vi "PrefDialog.vi"(8 "error in (no error)":errorcluster, 11 "MyPluginsBase in":refnum<class "NiDaqMx.lvclass">) -> (0 "error out":errorcluster, 3 "MyPluginsBase out":refnum<class "NiDaqMx.lvclass">)   [LabVIEW 2018, in "DigitizerPlugins.lvlib" / "NiDaqMx.lvclass"]
uses:
  NiDaqMx.lvclass
  X:/Projects/PMUCal/Modules/Digitizer/DigitizerPlugins/DigitizerBaseClass/DigitizerBase.lvclass
  C:/Program Files (x86)/National Instruments/LabVIEW 2018/user.lib/NIST/BaseClasses/BasePlugin_class/BasePlugin.lvclass
  DigitizerBaseClass/Typedefs/Acquisition.ctl
  DigitizerBaseClass/Typedefs/Channel.ctl
  DigitizerBaseClass/Typedefs/Trigger.ctl
  DigitizerBaseClass/Typedefs/TrigSource.ctl
  SampleClock.ctl
  Typedefs/Sync.ctl
  Typedefs/ExportSignal.ctl
  DigitizerBaseClass/DigitizerBase.lvclass/DigitizerBase.ctl
  NiDaqMx.lvclass/NiDaqMx.ctl
  <userlib>/NIST/BaseClasses/BasePlugin_class/BasePlugin.lvclass/BasePlugin.ctl
  DigitizerBaseClass/Accessors/Read Acquisition.vi
  DigitizerBaseClass/Accessors/Read Trigger.vi
  DigitizerBaseClass/Accessors/Read Channels.vi
  Accessors/Read SampleClock.vi
  Accessors/Read ExportSignal.vi
  DigitizerBaseClass/Accessors/Read SyncInfo.vi
  <userlib>/NIST/BaseClasses/BasePlugin_class/Accessors/Read PluginIniFilePath.vi
  DigitizerBaseClass/Accessors/Write Acquisition.vi
  DigitizerBaseClass/Accessors/Write Trigger.vi
  DigitizerBaseClass/Accessors/Write Channels.vi
  Accessors/Write SampleClock.vi
  DigitizerBaseClass/Accessors/Write SyncInfo.vi
  Accessors/Write ExportSignal.vi
  <userlib>/NIST/BaseClasses/BasePlugin_class/Accessors/Write PluginIniFilePath.vi
  <vilib>/Utility/config.llb/NI_LVConfig.lvlib
  DigitizerBaseClass/DigitizerBase.lvclass
panel:
  in  "cntrlTab":T1(tab)
  in  "Channels":T2[](array[typedef])
  in  "Acquisition":T3 {"SampleMode" items=["Real Time", "Equivalent Time"]}
  in  "Trigger":T4
  in  "ExportSignal":T6={"signal"=12487, "Destination"="none", "Route"="none"} {"signal" items=["AI Convert Clock"=12484, "10MHz Reference Clock"=12536, "20MHz Timebase Clock"=12486, "Sample Clock"=12487, "Advance Trigger"=12488, "Reference Trigger"=12490, "Start Trigger"=12491, "Advance Complete Event"=12492, "AI Hold Complete Event"=12493, "Counter Output Event"=12494, "Change Detection Event"=12511, "Watchdog Timer Expired Event"=12512]}
  in  "SampleClock":T7 {"sample mode" items=["Finite Samples"=10178, "Continuous Samples"=10123, "Hardware Timed Single Point"=12522]; "TimebaseRate" format="%#_6p"}
  in  "Sync":T8
  in  "btnSaveAs":bool
  in  "btnSave":bool
  in  "btnCancel":bool
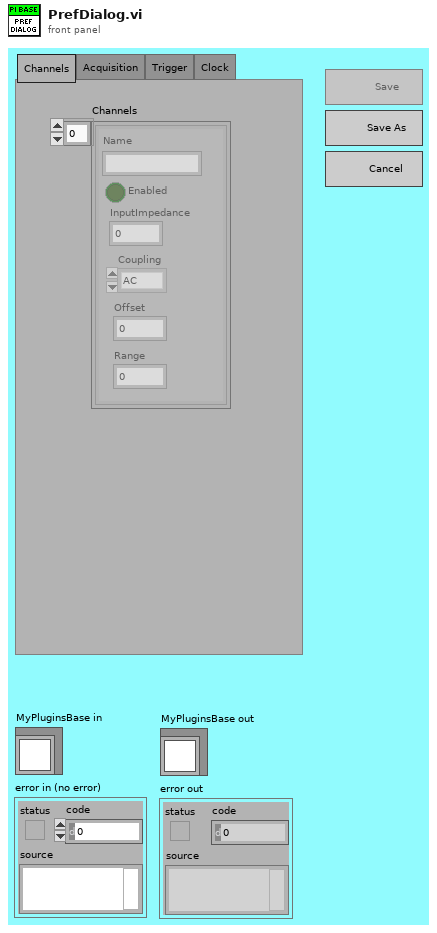
[diagram p1: front panel]
types:
  T1 = enum32{"Channels", "Acquisition", "Trigger", "Clock"}
  T2 = typedef "DigitizerPlugins.lvlib/DigitizerBase.lvclass/Channel.ctl" = cluster{"Name":string, "Enabled":bool, "InputImpedance":dbl, "Coupling":enum16{"AC", "DC", "Gnd"}, "Offset":dbl, "Range":dbl}
  T3 = typedef "DigitizerPlugins.lvlib/DigitizerBase.lvclass/Acquisition.ctl" = cluster{"SampleRate":dbl, "RecordSize":i32, "NumRecords":i32, "SampleMode":i32, "Timeout (ms)":i32}
  T4 = typedef "DigitizerPlugins.lvlib/DigitizerBase.lvclass/Trigger.ctl" = cluster{"Source":string, "Delay":dbl, "Holdoff":dbl, "PretriggerSamples":i32, "Sources":T5[]}
  T5 = typedef "DigitizerPlugins.lvlib/DigitizerBase.lvclass/TrigSource.ctl" = cluster{"Name":string, "Coupling":enum16{"AC", "DC", "HF Reject", "LF Reject", "Noise Reject"}, "Hysteresis":dbl, "Level":dbl, "Slope":enum16{"Positive", "Negative"}, "Type":enum16{"Edge", "Width", "Runt", "Glitch", "TV", "Window"}}
  T6 = typedef "DigitizerPlugins.lvlib/NiDaqMx.lvclass/ExportSignal.ctl" = cluster{"signal":i32, "Destination":string, "Route":string}
  T7 = typedef "DigitizerPlugins.lvlib/NiDaqMx.lvclass/SampleClock.ctl" = cluster{"Type":enum16{"NULL", "Onboard", "External", "Software", "Interval"}, "Source":string, "TimebaseRate":dbl, "sample mode":i32}
  T8 = typedef "DigitizerPlugins.lvlib/NiDaqMx.lvclass/Sync.ctl" = cluster{"Handle":string, "SrcTerm":string, "DestTerm":string}
  T9 = enum32{"Invalid", "Default", "Floating", "Floating/Auto-Hide", "Modal"}
  T10 = enum8{"Enabled", "Disabled", "Disabled and Grayed Out"}
  T11 = typedef "NI_LVConfig.lvlib/Config Data RefNum.ctl" = refnum<k1>
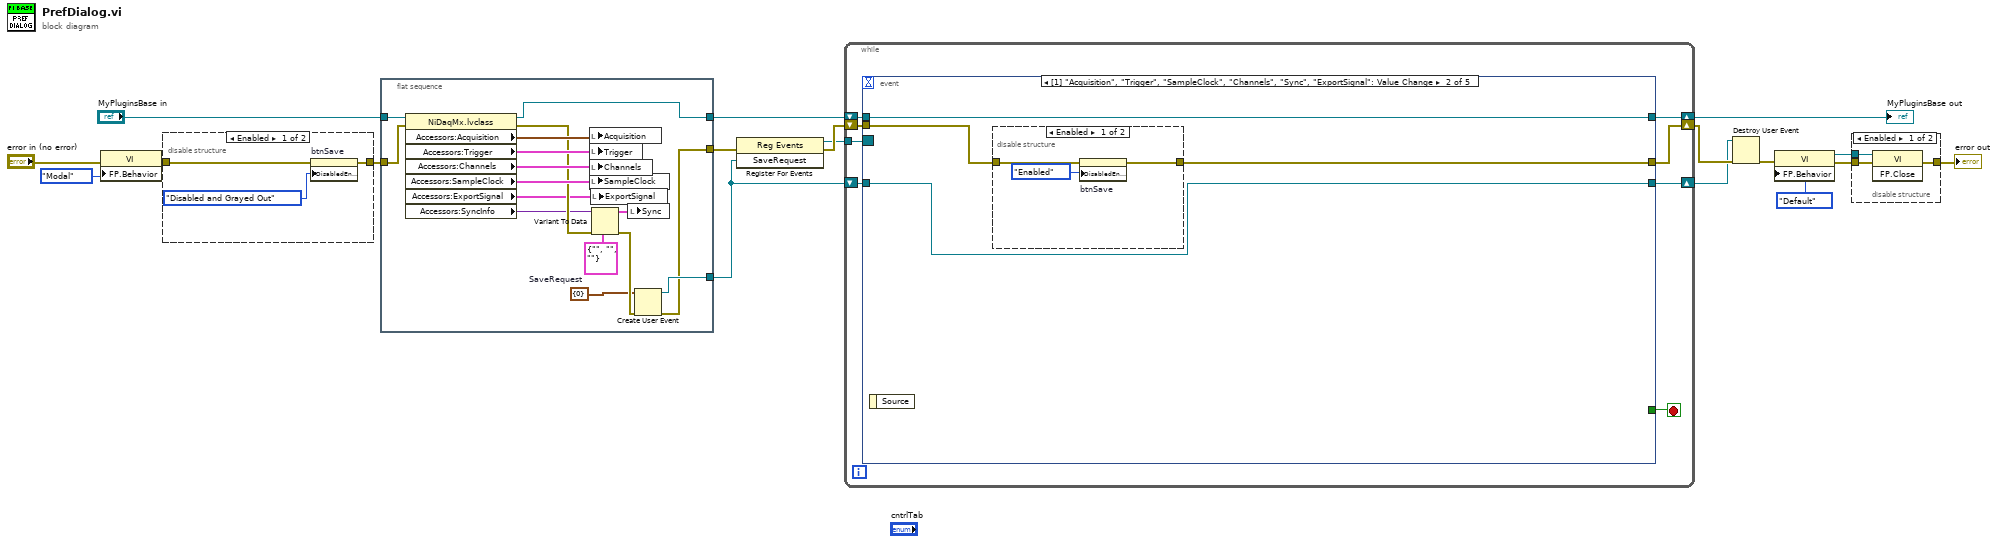
[diagram p0: block diagram]
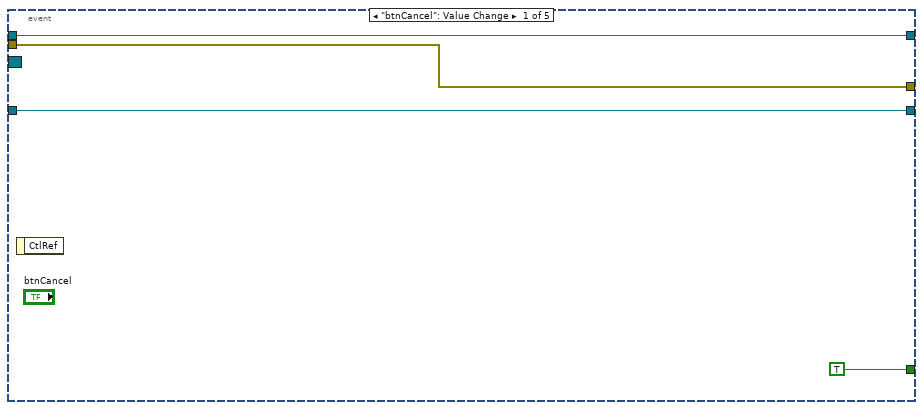
[diagram p4: hidden frame]
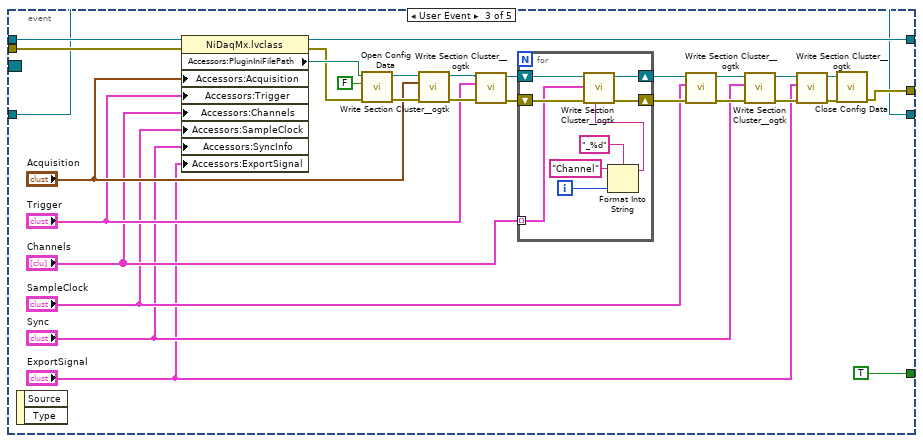
[diagram p6: hidden frame]
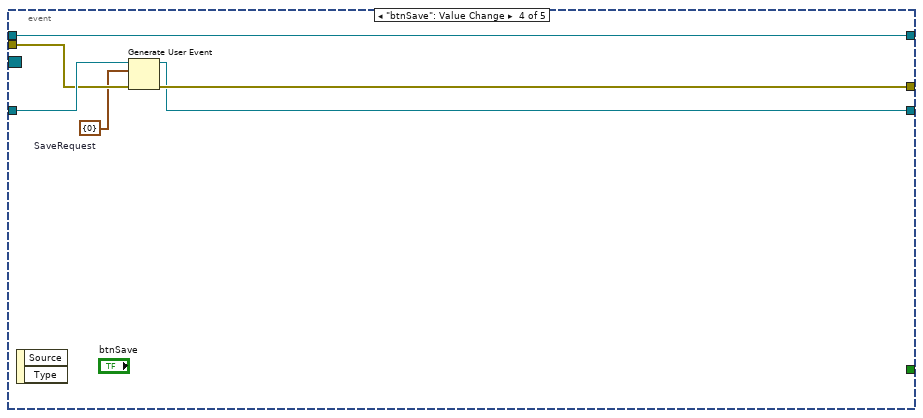
[diagram p7: hidden frame]
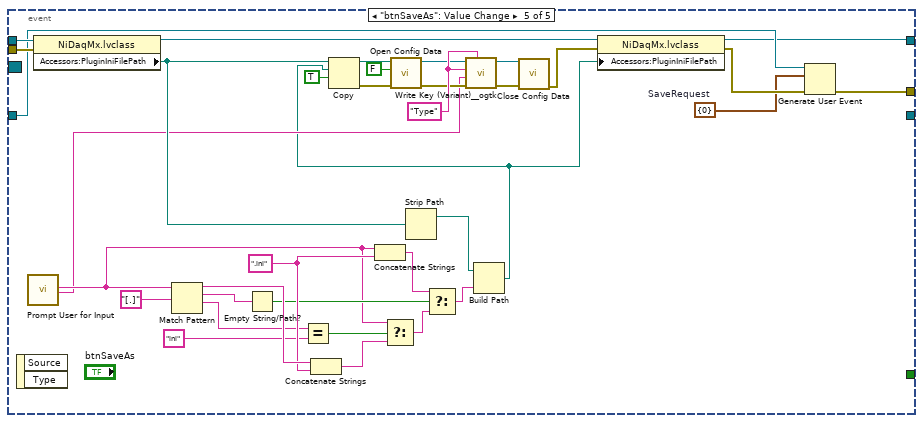
[diagram p8: hidden frame]
diagram:
  n1 = property class="VI"(error in="error in (no error)", "FP.Behavior"=T9."Modal" ("Front Panel Window:Behavior")) -> (error out=w9:errorcluster)  [unwired: 1 in, 1 out]
  n2 = disable-structure shown="Enabled" {
    disable-tunnel: w9 -> [w20 w22]
    disable-tunnel: [w19 w22] -> w8
    frame Enabled {
      n3 = property on="btnSave" class="Bool"(error in=w20, "DisabledEnum"=T10."Disabled and Grayed Out" ("Disabled")) -> (error out=w19:errorcluster)  [unwired: 1 in, 1 out]
    }
    frame Disabled {
    }
  }
  n4 = flat-sequence {
    tunnel: "MyPluginsBase in" -> [w38]
    tunnel: [w32] -> w10
    tunnel: [w25] -> w7
    tunnel: w8 -> [w30]
    tunnel: [w27] -> w2
    frame #0 {
      w24 = cluster{"num":i32} {"num"=0}  # SaveRequest
      n5 = property class="NiDaqMx.lvclass"(reference=w38, error in=w30) -> (reference out=w32:refnum<class "NiDaqMx.lvclass">, error out=w33:errorcluster, "Accessors:Acquisition"=w37:T3, "Accessors:Trigger"=w36:T4, "Accessors:Channels"=w35:T2[], "Accessors:SampleClock"=w34:T7, "Accessors:ExportSignal"=w23:T6, "Accessors:SyncInfo"=w31:variant)
      n6 = local write "Acquisition"(w37) -> ()
      n7 = local write "Trigger"(w36) -> ()
      n8 = local write "Channels"(w35) -> ()
      n9 = local write "SampleClock"(w34) -> ()
      n10 = local write "ExportSignal"(w23) -> ()
      n11 = Variant To Data(error in=w33, type=T8 {"Handle"="", "SrcTerm"="", "DestTerm"=""} ("Sync"), Variant=w31) -> (data=w28:T8, error out=w26:errorcluster)
      n12 = local write "Sync"(w28) -> ()
      n13 = Create User Event(user event datatype=w24, error in=w26) -> (user event=w27:refnum<user-event>, error out=w25:errorcluster)
    }
  }
  n14 = register-events(error in=w7, w2) -> (reference out=w5:refnum<event-registration>, error out=w6:errorcluster)  [unwired: 1 in]
  n15 = while {
    shift-right: [w46] -> w18
    shift-left: w10 -> [w44]
    shift-right: [w45] -> w3
    shift-left: w6 -> [w43]
    tunnel: w5 -> [w41]
    shift-right: [w39] -> w1
    shift-left: w2 -> [w40]
    stop <- w42 stop-if-true
    n16 = event shown="[1] \"Acquisition\", \"Trigger\", \"SampleClock\", \"Channels\", \"Sync\", \"ExportSignal\": Value Change" {
      selector: w41 -> [_ _ _ _ _]
      dyn-events: _ -> [_ _ _ _ _]
      timeout: _ -> [_ _ _ _ _]
      tunnel: w44 -> [w50 w54 w87 w98 w124]
      tunnel: [w50 w54 w74 w98 w103] -> w46
      tunnel: [w49 w52 w73 w99 w104] -> w45
      tunnel: w43 -> [w49 w53 w86 w101 w123]
      tunnel: [TRUE _ TRUE _ _] -> w42
      tunnel: w40 -> [w47 w51 w59 w102 w107]
      tunnel: [w47 w51 w59 w97 _] -> w39
      event "btnCancel": Value Change {
        n17 = event-data() -> ()  [unwired: 1 in, 1 out]
      }
      event "Channels": Value Change {
        n18 = event-data() -> ()  [unwired: 1 in, 1 out]
        n19 = disable-structure shown="Enabled" {
          disable-tunnel: w53 -> [w57 w58]
          disable-tunnel: [w56 w58] -> w52
          frame Enabled {
            n20 = property on="btnSave" class="Bool"(error in=w57, "DisabledEnum"=T10."Enabled" ("Disabled")) -> (error out=w56:errorcluster)  [unwired: 1 in, 1 out]
          }
          frame Disabled {
          }
        }
      }
      event User Event {
        n21 = event-data() -> ()  [unwired: 1 in, 2 out]
        n22 = property class="NiDaqMx.lvclass"(reference=w87, error in=w86, "Accessors:Acquisition"="Acquisition", "Accessors:Trigger"="Trigger", "Accessors:Channels"="Channels", "Accessors:SampleClock"="SampleClock", "Accessors:SyncInfo"="Sync", "Accessors:ExportSignal"="ExportSignal") -> (reference out=w74:refnum<class "NiDaqMx.lvclass">, error out=w83:errorcluster, "Accessors:PluginIniFilePath"=w85:path)
        n23 = call <vilib>:"Open Config Data.vi"("error in (no error)"=w83, "create file if necessary (T)"=FALSE, "configuration file path"=w85) -> ("error out"=w81:errorcluster, "refnum"=w82:T11)  [unwired: 6 in, 1 out]
        n24 = call <userlib>:"Write Section Cluster__ogtk.vi"("error in (no error)"=w81, "Section Formatted Cluster"="Acquisition", "refnum"=w82) -> ("error out"=w79:errorcluster, "dup refnum"=w80:T11)  [unwired: 7 in]
        n25 = call <userlib>:"Write Section Cluster__ogtk.vi"("error in (no error)"=w79, "Section Formatted Cluster"="Trigger", "refnum"=w80) -> ("error out"=w78:errorcluster, "dup refnum"=w77:T11)  [unwired: 7 in]
        n26 = for {
          shift-right: [w94] -> w76
          shift-left: w78 -> [w96]
          shift-right: [w93] -> w75
          shift-left: w77 -> [w95]
          tunnel: "Channels" -> [w89] mode=indexing
          i -> [w90]
          n27 = Format Into String(format string="_%d", initial string="Channel", w90) -> (resulting string=w88:string)  [unwired: 1 in, 1 out]
          n28 = call <userlib>:"Write Section Cluster__ogtk.vi"("section (optional)"=w88, "error in (no error)"=w96, "Section Formatted Cluster"=w89, "refnum"=w95) -> ("error out"=w94:errorcluster, "dup refnum"=w93:T11)  [unwired: 6 in]
        }
        n29 = call <userlib>:"Write Section Cluster__ogtk.vi"("error in (no error)"=w76, "Section Formatted Cluster"="SampleClock", "refnum"=w75) -> ("error out"=w68:errorcluster, "dup refnum"=w67:T11)  [unwired: 7 in]
        n30 = call <userlib>:"Write Section Cluster__ogtk.vi"("error in (no error)"=w68, "Section Formatted Cluster"="Sync", "refnum"=w67) -> ("error out"=w62:errorcluster, "dup refnum"=w61:T11)  [unwired: 7 in]
        n31 = call <userlib>:"Write Section Cluster__ogtk.vi"("error in (no error)"=w62, "Section Formatted Cluster"="ExportSignal", "refnum"=w61) -> ("error out"=w64:errorcluster, "dup refnum"=w63:T11)  [unwired: 7 in]
        n32 = call <vilib>:"Close Config Data.vi"("error in (no error)"=w64, "refnum"=w63) -> ("error out"=w73:errorcluster)  [unwired: 8 in, 1 out]
      }
      event "btnSave": Value Change {
        w100 = cluster{i32} {0}  # SaveRequest
        n33 = event-data() -> ()  [unwired: 1 in, 2 out]
        n34 = Generate User Event(user event=w102, event data cluster=w100, error in=w101) -> (user event out=w97:refnum<user-event>, error out=w99:errorcluster)  [unwired: 1 in]
      }
      event "btnSaveAs": Value Change {
        w105 = cluster{i32} {0}  # SaveRequest
        w120 = "Type" ("key (optional)")
        w135 = ".ini" ("string")
        n35 = event-data() -> ()  [unwired: 1 in, 2 out]
        n36 = call "Prompt User for Input"() -> ("File Name"=w126:string, "PluginType"=w111:string)  [unwired: 16 in, 2 out]
        n37 = property class="NiDaqMx.lvclass"(reference=w124, error in=w123) -> (reference out=w110:refnum<class "NiDaqMx.lvclass">, "Accessors:PluginIniFilePath"=w113:path)  [unwired: 1 out]
        n38 = Match Pattern(string=w126, regular expression="[.]" ("string")) -> (before substring=w136:string, match substring=w132:string, after substring=w133:string)  [unwired: 1 in, 1 out]
        n39 = Empty String/Path?(string/path=w132) -> (empty?=w127:bool)
        n40 = Equal?(x=w133, y="ini" ("string")) -> (x = y?=w129:bool)
        n41 = Concatenate Strings(w136, w135) -> (w137:string)
        n42 = Concatenate Strings(w126, w135) -> (w128:string)
        n43 = Select(t=w126, s=w129, f=w137) -> (s? t:f=w130:string)
        n44 = Strip Path(path=w113) -> (stripped path=w112:path)  [unwired: 1 out]
        n45 = Select(t=w128, s=w127, f=w130) -> (s? t:f=w125:string)
        n46 = Build Path(base path=w112, name or relative path=w125) -> (appended path=w109:path)
        n47 = Copy(9:TRUE ("overwrite (F)"), 10:w109, 11:w113) -> (0:w117:errorcluster, 3:w116:path)  [unwired: 2 in, 1 out]
        n48 = call <vilib>:"Open Config Data.vi"("error in (no error)"=w117, "create file if necessary (T)"=FALSE, "configuration file path"=w116) -> ("error out"=w118:errorcluster, "refnum"=w119:T11)  [unwired: 6 in, 1 out]
        n49 = call <userlib>:"Write Key (Variant)__ogtk.vi"("section"=w120, "error in (no error)"=w118, "key-value"=w111, "key (optional)"=w120, "refnum"=w119) -> ("error out"=w122:errorcluster, "refnum out"=w121:T11)  [unwired: 5 in]
        n50 = call <vilib>:"Close Config Data.vi"("error in (no error)"=w122, "refnum"=w121) -> ("error out"=w108:errorcluster)  [unwired: 8 in, 1 out]
        n51 = property class="NiDaqMx.lvclass"(reference=w110, error in=w108, "Accessors:PluginIniFilePath"=w109) -> (reference out=w103:refnum<class "NiDaqMx.lvclass">, error out=w106:errorcluster)
        n52 = Generate User Event(user event=w107, event data cluster=w105, error in=w106) -> (error out=w104:errorcluster)  [unwired: 1 in, 1 out]
      }
    }
  }
  "MyPluginsBase out" <- w18
  n53 = Destroy User Event(user event=w1, error in=w3) -> (error out=w4:errorcluster)
  n54 = property class="VI"(error in=w4, "FP.Behavior"=T9."Default" ("Front Panel Window:Behavior")) -> (reference out=w13:refnum<vi>, error out=w16:errorcluster)  [unwired: 1 in]
  n55 = disable-structure shown="Enabled" {
    disable-tunnel: w16 -> [w140 w141]
    disable-tunnel: [w139 w141] -> w14
    disable-tunnel: w13 -> [w138 _]
    frame Enabled {
      n56 = invoke class="VI" method="FP.Close"(reference=w138, error in=w140) -> (error out=w139:errorcluster)  [unwired: 1 in, 2 out]
    }
    frame Disabled {
    }
  }
  "error out" <- w14
